vi "MakeColdLoopCode.vi"(11 "ColdPWM":dbl=-30.0 min=-230.0 max=30.0) -> (3 "resulting string":string)   [LabVIEW 2023]
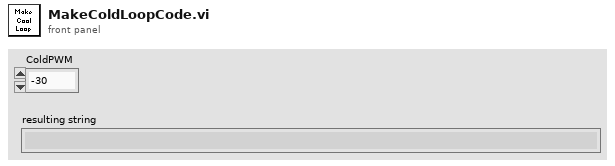
[diagram p1: front panel]
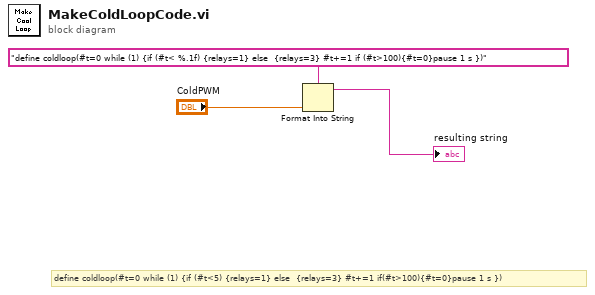
[diagram p0: block diagram]
diagram:
  # "define coldloop(#t=0 while (1) {if (#t<5) {relays=1} else  {relays=3} #t+=1 if(#t>100){#t=0}pause 1 s })"
  n1 = Format Into String(format string="define coldloop(#t=0 while (1) {if (#t< %.1f) {relays=1} else  {relays=3} #t+=1 if (#t>100){#t=0}pause 1 s })", "ColdPWM") -> (resulting string=→"resulting string":string)  [unwired: 2 in, 1 out]
